vi "ExGetCustomTiming.vi"(1 "error in (no error)":errorcluster, 2 "vertical timing index":dbl=1.0) -> (0 "error out":errorcluster)   [LabVIEW 2010]
uses:
  Open-Close Hardware/CamHandle.vi
panel:
  out "Enum Information":T1 {"Enum Value" format="%.2f"}
  # "ExCustomTiming.vi :"
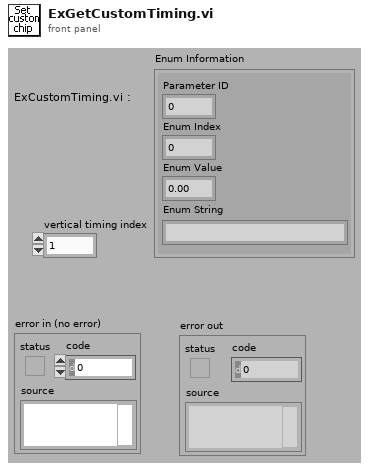
[diagram p1: front panel]
types:
  T1 = cluster{"Parameter ID":u32, "Enum Index":u32, "Enum Value":dbl, "Enum String":string}
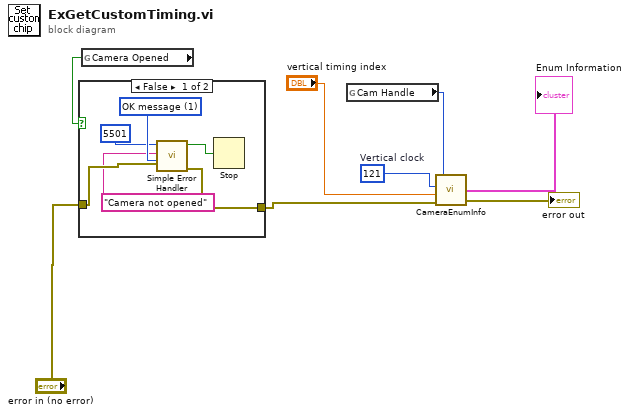
[diagram p0: block diagram]
diagram:
  w3 = u32 121  # Vertical clock
  n1 = global read "CamHandle.vi" "Camera Opened"() -> (w8:bool)
  n2 = case shown="False" w8 {
    tunnel: "error in (no error)" -> [w13 w15]
    tunnel: [w12 w15] -> w6
    frame False {
      w14 = u16 1 items=["no dialog", "OK message", "continue or stop message"] ("type of dialog (OK msg:1)")
      n3 = call <vilib>:"Simple Error Handler.vi"("error code (no error:0)"=5501, "error source (\" \")"="Camera not opened", "type of dialog (OK msg:1)"=w14, "error in (no error)"=w13) -> ("error?"=w10:bool, "error out"=w12:errorcluster)  [unwired: 1 in, 3 out]
      n4 = Stop(stop? (T)=w10) -> ()
    }
    frame True {
    }
  }
  n5 = global read "CamHandle.vi" "Cam Handle"() -> (w1:u32)
  n6 = call <userlib>:"CameraEnumInfo.vi"("error in"=w6, "Enum Index"="vertical timing index", "Parameter ID"=w3, "Camera Handle"=w1) -> ("error out"=→"error out":errorcluster, "Enum Information"=→"Enum Information":T1)  [unwired: 1 out]
